vi "Insert Plugin - Splash.vi"(10 "Message Queues":T1, 11 "SubPanel in":refnum<vi>) -> (0 "error out":errorcluster, 3 "VI out":refnum<vi>)   [LabVIEW 2019]
uses:
  support/Copy of Message Queue/All Message Queues.ctl
  support/Copy of Message Queue/Message Cluster.ctl
  support/Copy of Message Queue/Copy of Message Queue.lvlib
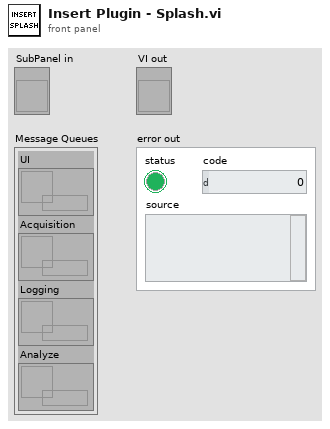
[diagram p1: front panel]
types:
  T1 = typedef "Copy of Message Queue.lvlib/All Message Queues.ctl" = cluster{"UI":refnum<queue>, "Acquisition":refnum<queue>, "Logging":refnum<queue>, "Analyze":refnum<queue>}
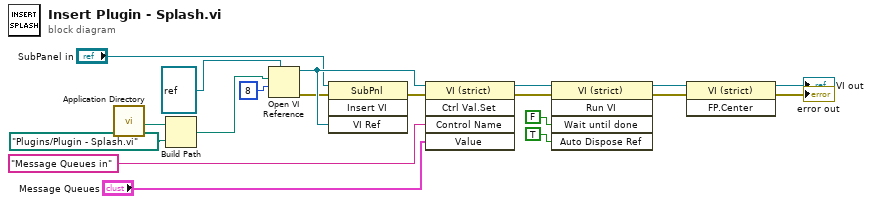
[diagram p0: block diagram]
diagram:
  n1 = call <vilib>:"Application Directory.vi"() -> ("Application Directory"=w1:path)
  n2 = Build Path(base path=w1, name or relative path=path "Plugins/Plugin - Splash.vi" ("vi path")) -> (appended path=w3:path)
  n3 = Open VI Reference(type specifier VI Refnum (for type only)=refnum<vi> refnum ("reference out"), vi path=w3, options=8) -> (vi reference=w14:refnum<vi>, error out=w8:errorcluster)  [unwired: 3 in]
  n4 = invoke on="Invoke Node" class="SubPnl" method="Insert VI"(reference="SubPanel in", error in=w8, "VI Ref"=w14) -> (error out=w15:errorcluster)  [unwired: 1 in, 3 out]
  n5 = invoke class="VI (strict)" method="Ctrl Val.Set"(reference=w14, error in=w15, "Control Name"="Message Queues in", "Value"="Message Queues") -> (reference out=w16:refnum<vi>, error out=w19:errorcluster)  [unwired: 1 in, 3 out]
  n6 = invoke class="VI (strict)" method="Run VI"(reference=w16, error in=w19, "Wait until done"=FALSE ("Wait Until Done"), "Auto Dispose Ref"=TRUE ("Wait Until Done")) -> (reference out=w17:refnum<vi>, error out=w18:errorcluster)  [unwired: 1 in, 3 out]
  n7 = invoke class="VI (strict)" method="FP.Center"(reference=w17, error in=w18) -> (reference out=→"VI out":refnum<vi>, error out=→"error out":errorcluster)  [unwired: 1 in, 1 out]
